vi "主程序.vi"() -> ()   [LabVIEW 2012]
panel:
  out "数组":u32[][](array[colorbox])
  in  "状态 2":bool=TRUE
  in  "得分":dbl
  out "难度":dbl
  in  "状态":bool=TRUE
  in  "ID":i8
  in  "偏移量":cluster{"X":i32, "Y":i32}
  # "显示区"
  # "额外信息"
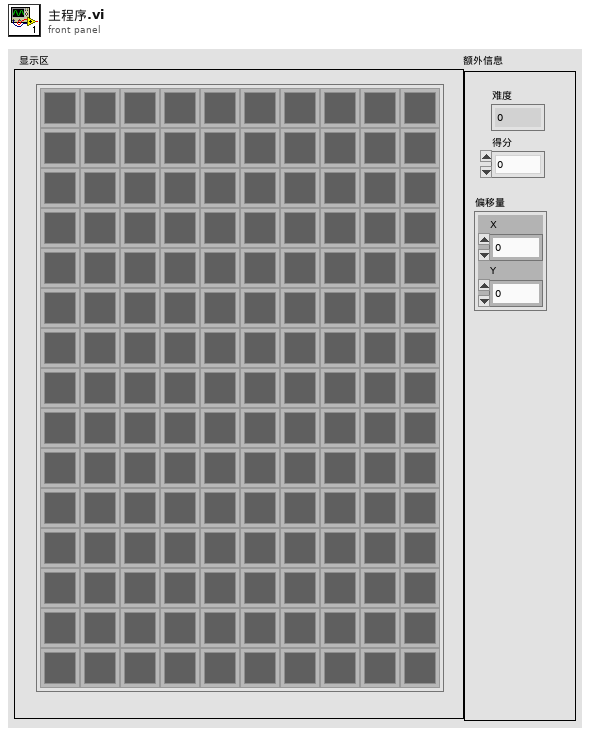
[diagram p1: front panel]
types:
  T1 = typedef "eventvkey.ctl" = enum16{"ASCII", "Enter", "Return", "Shift", "Ctrl", "Alt", "Cmd", "Opt", "Caps", "NumLock", "Clear", "Break", "Up", "Down", "Left", "Right", "Insert", "Delete", "Home", "End", "PageUp", "PageDown", "Escape", "Help", "Pause", "ScrollLock", "F1", "F2", "F3", "F4", "F5", "F6", "F7", "F8", "F9", "F10", "F11", "F12", "F13", "F14", "F15", "F16", "F17", "F18", "F19", "F20", "F21", "F22", "F23", "F24", "Play", "VolumeUp", "VolumeDown", "Mute", "Two Byte Char"}
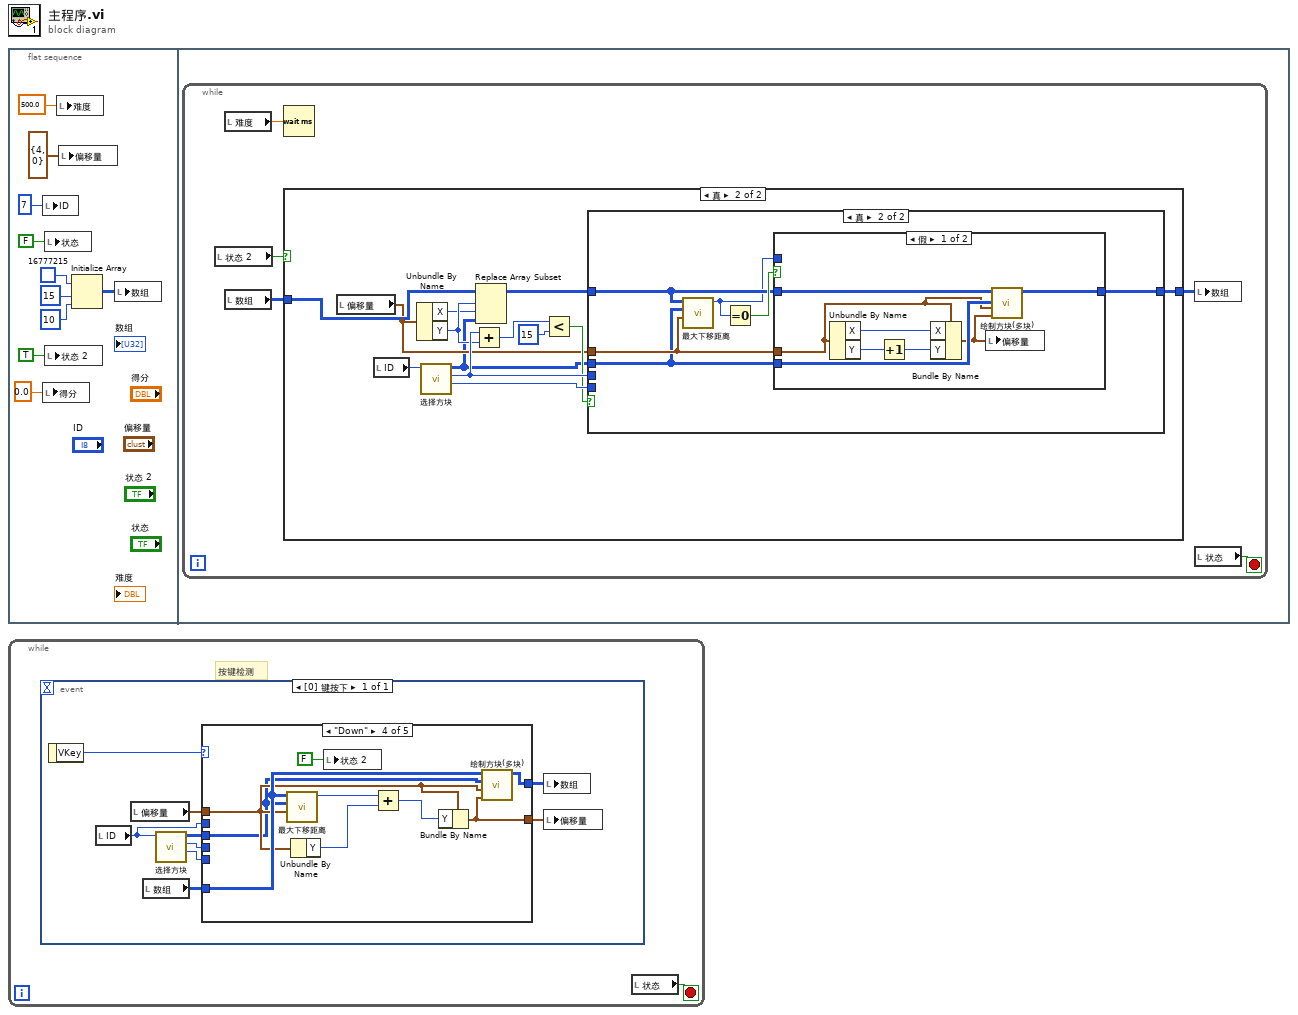
[diagram p0: block diagram]
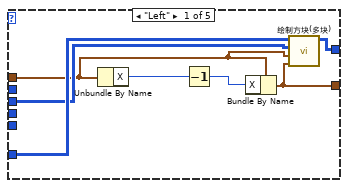
[diagram p2: hidden frame]
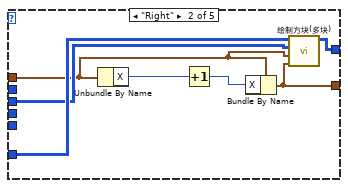
[diagram p3: hidden frame]
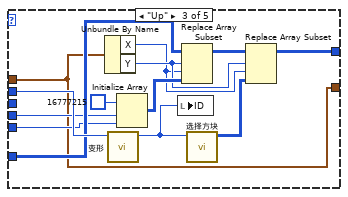
[diagram p4: hidden frame]
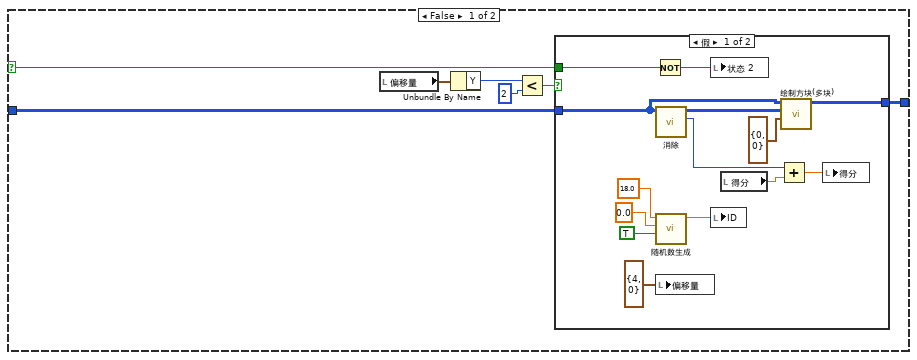
[diagram p6: hidden frame]
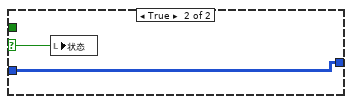
[diagram p7: hidden frame]
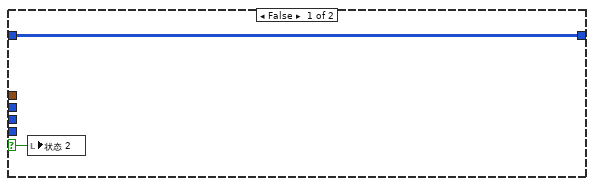
[diagram p8: hidden frame]
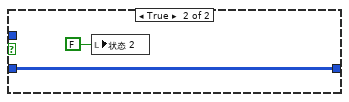
[diagram p9: hidden frame]
diagram:
  n1 = flat-sequence {
    frame #0 {
      n2 = local write "ID"(i8 7 ("ID")) -> ()
      n3 = local write "得分"(0.0 ("得分")) -> ()
      n4 = local write "状态"(FALSE ("状态")) -> ()
      n5 = local write "状态 2"(TRUE ("状态 2")) -> ()
      n6 = local write "难度"(500.0 ("难度")) -> ()
      n7 = local write "偏移量"(cluster{"X":i32, "Y":i32} {"X"=4, "Y"=0} ("偏移量")) -> ()
      n8 = Initialize Array(u32 16777215, 15 ("维数大小"), 10 ("维数大小")) -> (w7:u32[][])
      n9 = local write "数组"(w7) -> ()
    }
    frame #1 {
      n10 = while {
        stop <- w15 stop-if-true
        n11 = local read "状态 2"() -> (w14:bool)
        n12 = local read "难度"() -> (w11:dbl)
        n13 = local read "数组"() -> (w13:u32[][])
        n14 = Wait (ms)(milliseconds to wait=w11) -> ()  [unwired: 1 out]
        n15 = case shown="真" w14 {
          selector: w14 -> [w20 _]
          tunnel: w13 -> [w21 w50]
          tunnel: [w22 w48] -> w12
          frame False {
            n16 = local read "偏移量"() -> (w19:cluster{"X":i32, "Y":i32})
            n17 = Unbundle By Name(w19) -> ("Y"=w17:i32)
            n18 = Less?(x=w17, y=2) -> (x < y?=w18:bool)
            n19 = case shown="假" w18 {
              selector: w18 -> [_ w38]
              tunnel: [w23 w37] -> w22
              tunnel: w21 -> [w26 w37]
              tunnel: w20 -> [w28 _]
              frame False {
                n20 = Not(x=w28) -> (.not. x?=w27:bool)
                n21 = call "消除.vi"("数组"=w26) -> ("得分"=w31:i8, "数组 2"=w25:u32[][])  [unwired: 9 in]
                n22 = call "随机数生成.vi"("整数/浮点"=TRUE, "下限"=0.0, "上限"=18.0) -> ("输出"=w34:dbl)  [unwired: 8 in]
                n23 = local write "偏移量"(cluster{"X":i32, "Y":i32} {"X"=4, "Y"=0} ("偏移量")) -> ()
                n24 = local write "状态 2"(w27) -> ()
                n25 = local write "ID"(w34) -> ()
                n26 = local read "得分"() -> (w32:dbl)
                n27 = Add(x=w31, y=w32) -> (x+y=w30:dbl)
                n28 = call "绘制方块(多块).vi"("偏移量"=cluster{"X":i32, "Y":i32} {"X"=0, "Y"=0}, "数组 2"=w25, "数组"=w26) -> ("数组 3"=w23:u32[][])  [unwired: 8 in]
                n29 = local write "得分"(w30) -> ()
              }
              frame True {
                n30 = local write "状态"(w38) -> ()
              }
            }
          }
          frame True {
            n31 = local read "偏移量"() -> (w43:cluster{"X":i32, "Y":i32})
            n32 = local read "ID"() -> (w51:i8)
            n33 = Unbundle By Name(w43) -> ("X"=w40:i32, "Y"=w41:i32)
            n34 = call "选择方块.vi"("ID"=w51) -> ("列"=w49:i32, "行"=w47:i32, "数组"=w39:u32[][])  [unwired: 8 in]
            n35 = Add(x=w47, y=w41) -> (x+y=w46:i32)
            n36 = Replace Array Subset(array=w50, new element=w39, index (row)=w41, index (col)=w40) -> (w42:u32[][])
            n37 = Less?(x=w46, y=15) -> (x < y?=w44:bool)
            n38 = case shown="真" w44 {
              selector: w44 -> [w52 _]
              tunnel: w42 -> [w53 w58]
              tunnel: w39 -> [_ w54]
              tunnel: w49 -> [_ _]
              tunnel: [w53 w57] -> w48
              tunnel: w47 -> [_ _]
              tunnel: w43 -> [_ w55]
              frame False {
                n39 = local write "状态 2"(w52) -> ()
              }
              frame True {
                n40 = call "最大下移距离.vi"("偏移量"=w55, "数组 2"=w54, "数组"=w58) -> ("最大下移距离"=w56:i32)  [unwired: 8 in]
                n41 = Equal To 0?(x=w56) -> (x = 0?=w59:bool)
                n42 = case shown="假" w59 {
                  tunnel: w58 -> [w64 w68]
                  tunnel: [w60 w68] -> w57
                  tunnel: w56 -> [_ _]
                  tunnel: w55 -> [w62 _]
                  tunnel: w54 -> [w63 _]
                  frame False {
                    n43 = Unbundle By Name(w62) -> ("X"=w67:i32, "Y"=w66:i32)
                    n44 = Increment(x=w66) -> (x+1=w65:i32)
                    n45 = Bundle By Name(cluster=w62, "X"=w67, "Y"=w65) -> (w61:cluster{"X":i32, "Y":i32})
                    n46 = local write "偏移量"(w61) -> ()
                    n47 = call "绘制方块(多块).vi"("偏移量 2"=w61, "偏移量"=w62, "数组 2"=w63, "数组"=w64) -> ("数组 3"=w60:u32[][])  [unwired: 7 in]
                  }
                  frame True {
                    n48 = local write "状态 2"(FALSE ("状态 2")) -> ()
                  }
                }
              }
            }
          }
        }
        n49 = local write "数组"(w12) -> ()
        n50 = local read "状态"() -> (w15:bool)
      }
    }
  }
  n51 = while {
    stop <- w70 stop-if-true
    # "按键检测"
    n52 = event shown="[0] 键按下" {
      selector: _ -> [_]
      dyn-events: _ -> [_]
      timeout: _ -> [_]
      event Key Down {
        n53 = event-data() -> ("VKey"=w79:T1)  [unwired: 1 in]
        n54 = local read "ID"() -> (w73:i8)
        n55 = local read "偏移量"() -> (w78:cluster{"X":i32, "Y":i32})
        n56 = local read "数组"() -> (w76:u32[][])
        n57 = call "选择方块.vi"("ID"=w73) -> ("列"=w71:i32, "行"=w72:i32, "数组"=w74:u32[][])  [unwired: 8 in]
        n58 = case shown="\"Down\"" w79 {
          tunnel: w78 -> [w81 w89 w99 w108 w116]
          tunnel: [w80 w88 w99 w109 w116] -> w77
          tunnel: w76 -> [w84 w91 w105 w111 w117]
          tunnel: [w82 w87 w94 w110 w117] -> w75
          tunnel: w74 -> [w83 w90 _ w107 _]
          tunnel: w72 -> [_ _ w102 _ _]
          tunnel: w71 -> [_ _ w103 _ _]
          tunnel: w73 -> [_ _ w106 _ _]
          frame "Left" {
            n59 = Unbundle By Name(w81) -> ("X"=w86:i32)
            n60 = Decrement(x=w86) -> (x-1=w85:i32)
            n61 = Bundle By Name(cluster=w81, "X"=w85) -> (w80:cluster{"X":i32, "Y":i32})
            n62 = call "绘制方块(多块).vi"("偏移量 2"=w80, "偏移量"=w81, "数组 2"=w83, "数组"=w84) -> ("数组 3"=w82:u32[][])  [unwired: 7 in]
          }
          frame "Right" {
            n63 = Unbundle By Name(w89) -> ("X"=w93:i32)
            n64 = Increment(x=w93) -> (x+1=w92:i32)
            n65 = Bundle By Name(cluster=w89, "X"=w92) -> (w88:cluster{"X":i32, "Y":i32})
            n66 = call "绘制方块(多块).vi"("偏移量 2"=w88, "偏移量"=w89, "数组 2"=w90, "数组"=w91) -> ("数组 3"=w87:u32[][])  [unwired: 7 in]
          }
          frame "Up" {
            n67 = Unbundle By Name(w99) -> ("X"=w95:i32, "Y"=w96:i32)
            n68 = call "变形.vi"("数值"=w106) -> ("数值 2"=w104:i8)  [unwired: 10 in]
            n69 = Initialize Array(u32 16777215, w102, w103) -> (w100:u32[][])
            n70 = local write "ID"(w104) -> ()
            n71 = Replace Array Subset(array=w105, new element=w100, index (row)=w96, index (col)=w95) -> (w97:u32[][])
            n72 = call "选择方块.vi"("ID"=w104) -> ("数组"=w98:u32[][])  [unwired: 8 in, 2 out]
            n73 = Replace Array Subset(array=w97, new element=w98, index (row)=w96, index (col)=w95) -> (w94:u32[][])
          }
          frame "Down" {
            n74 = call "最大下移距离.vi"("偏移量"=w108, "数组 2"=w107, "数组"=w111) -> ("最大下移距离"=w114:i32)  [unwired: 8 in]
            n75 = Unbundle By Name(w108) -> ("Y"=w115:i32)
            n76 = local write "状态 2"(FALSE ("状态 2")) -> ()
            n77 = Add(x=w114, y=w115) -> (x+y=w113:i32)
            n78 = Bundle By Name(cluster=w108, "Y"=w113) -> (w109:cluster{"X":i32, "Y":i32})
            n79 = call "绘制方块(多块).vi"("偏移量 2"=w109, "偏移量"=w108, "数组 2"=w107, "数组"=w111) -> ("数组 3"=w110:u32[][])  [unwired: 7 in]
          }
          frame "Insert", Default {
          }
        }
        n80 = local write "数组"(w75) -> ()
        n81 = local write "偏移量"(w77) -> ()
      }
    }
    n82 = local read "状态"() -> (w70:bool)
  }
